vi "Acquisition Module.vi"(8 "Error In":errorcluster, 11 "Queues Cluster":T1) -> (0 "Error Out":errorcluster)   [LabVIEW 2017]
uses:
  Typedefs/Imaging Protocols enum.ctl
  User Interface/Queue/Message Queue/Typedefs/All Message Queues.ctl
  User Interface/Queue/Message Queue/Typedefs/Message Cluster.ctl
  Typedefs/Logging queue element.ctl
  Typedefs/Frame Size.ctl
  Typedefs/Acquired points count.ctl
  Video Rec Signaling/typedefs/Functions enum.ctl
  Typedefs/Read Write Enum.ctl
  Global Variables/General Globals.vi
panel:
  out "Rate":u32
  out "Acq":u32
  out "Start":u32
  out "?":errorcluster
  out "Imaging Protocol":T2=enum."Live Imaging"
  out "Acquired z-plane index":i32
  out "State":string
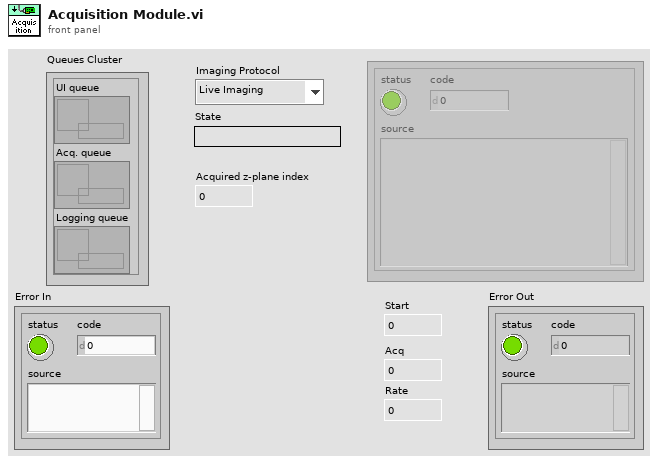
[diagram p1: front panel]
types:
  T1 = typedef "All Message Queues.ctl" = cluster{"UI queue":refnum<queue>, "Acq. queue":refnum<queue>, "Logging queue":refnum<queue>}
  T2 = typedef "Imaging Protocols enum.ctl" = enum16{"AOL Z-Stack", "Motor Z Stack", "Functional Acquisition", "Single Plane Acquisition", "Volume Acquisition", "Live Imaging", "Live Plane Imaging", "Live Volume Imaging"}
  T3 = typedef "Functions enum.ctl" = enum16{"Create", "Start", "Write", "Stop", "Clear"}
  T4 = enum8{"Enabled", "Disabled", "Disabled and Grayed Out"}
  T5 = typedef "Read Write Enum.ctl" = enum16{"Read", "Write"}
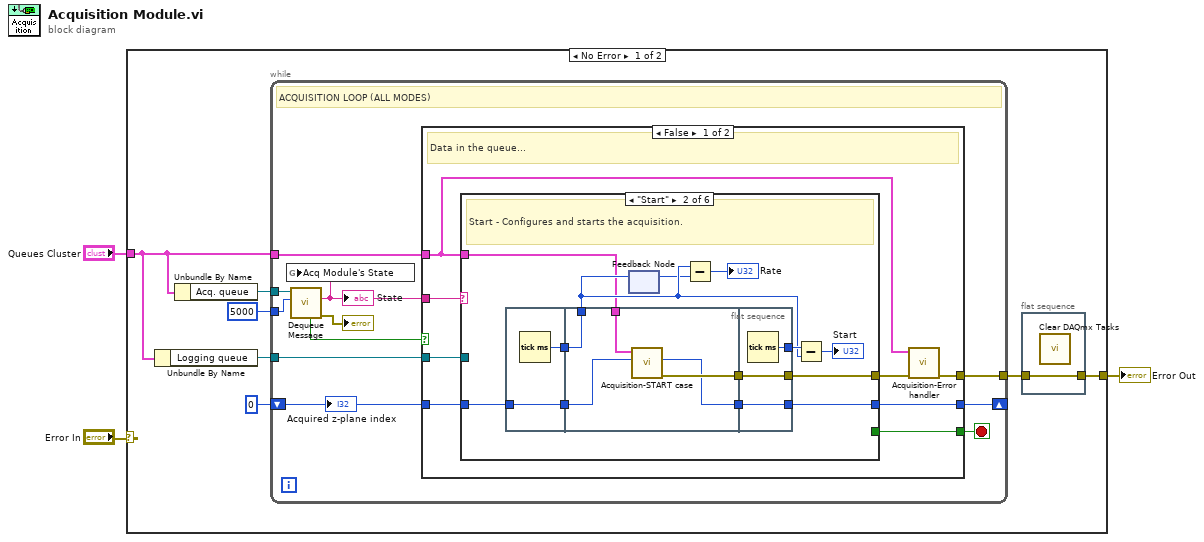
[diagram p0: block diagram]
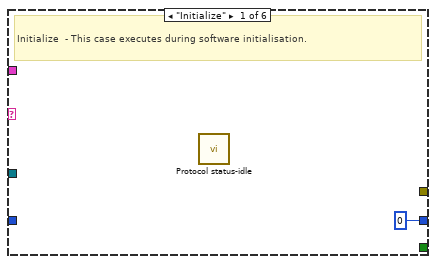
[diagram p2: hidden frame]
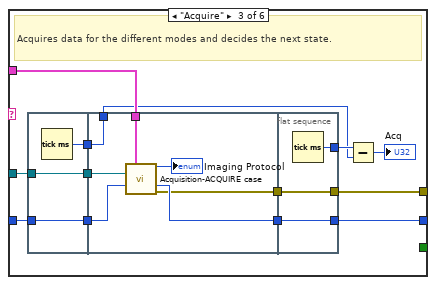
[diagram p3: hidden frame]
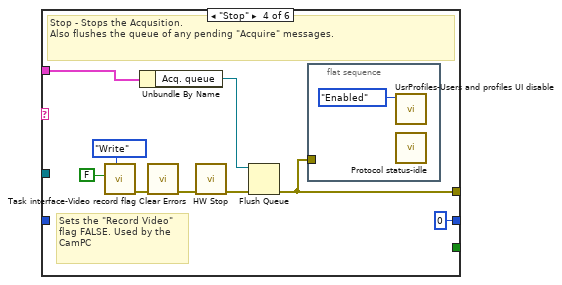
[diagram p4: hidden frame]
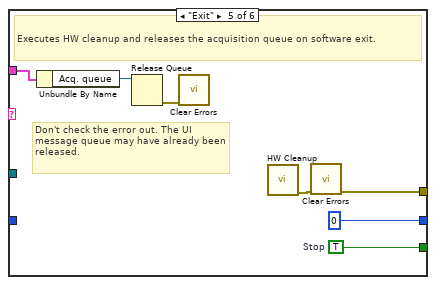
[diagram p5: hidden frame]
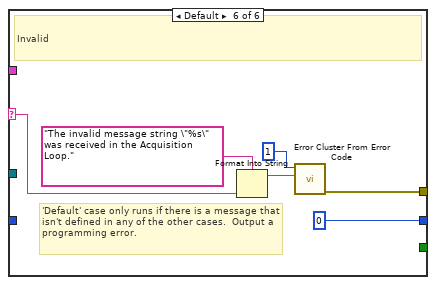
[diagram p6: hidden frame]
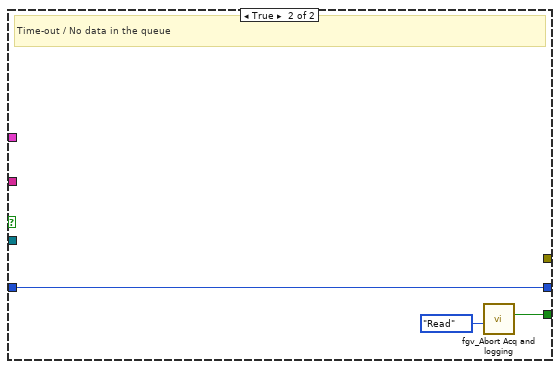
[diagram p7: hidden frame]
diagram:
  n1 = case shown="No Error" "Error In" {
    selector: "Error In" -> [_ w107]
    tunnel: "Queues Cluster" -> [w6 _]
    tunnel: [w7 w107] -> w2
    frame No Error {
      n2 = Unbundle By Name(w6) -> ("Logging queue"=w5:refnum<queue>)
      n3 = Unbundle By Name(w6) -> ("Acq. queue"=w10:refnum<queue>)
      n4 = while {
        tunnel: w10 -> [w19]
        tunnel: w5 -> [w21]
        shift-right: [w20] -> _
        shift-left: 0 -> [w18]
        tunnel: w6 -> [w17]
        tunnel: [w15] -> w8
        tunnel: 5000 ("timeout in ms (-1)") -> [w14]
        stop <- w22 stop-if-true
        # "ACQUISITION LOOP (ALL MODES)"
        n5 = call "Dequeue Message.vi"("timeout in ms (-1)"=w14, "Message Queue"=w19) -> ("Error Out"=→"?":errorcluster, "Message"=w12:string, "timed out?"=w13:bool)  [unwired: 5 in, 2 out]
        "State" <- w12
        n6 = global write "General Globals.vi" "Acq Module's State"(w12) -> ()
        n7 = case shown="False" w13 {
          tunnel: [w30 w104] -> w22
          tunnel: w21 -> [w29 _]
          tunnel: [w28 w106] -> w20
          tunnel: w18 -> [w27 w106]
          tunnel: w12 -> [w25 _]
          tunnel: w17 -> [w23 _]
          tunnel: [w24 _] -> w15
          frame False {
            # "Data in the queue..."
            n8 = case "Message Cases" shown="\"Start\"" w25 {
              selector: w25 -> [_ _ _ _ _ w99]
              tunnel: [_ w44 w64 w81 w91 w101] -> w26
              tunnel: [_ _ _ _ w97 _] -> w30
              tunnel: w29 -> [_ _ w67 _ _ _]
              tunnel: w27 -> [_ w43 w63 _ _ _]
              tunnel: [0 ("Index of next Z-plane to acquire") w42 w66 0 ("Index of next Z-plane to acquire") 0 ("Index of next Z-plane to acquire") 0 ("Index of next Z-plane to acquire")] -> w28
              tunnel: w23 -> [_ w32 w65 w82 w95 _]
              frame "Initialize" {
                # "Initialize  - This case executes during software initialisation."
                n9 = call "Protocol status-idle.vi"() -> ()  [unwired: 12 in]
              }
              frame "Start" {
                # "Start - Configures and starts the acquisition."
                n10 = flat-sequence {
                  tunnel: w43 -> [w46]
                  tunnel: [w46] -> w39
                  tunnel: [w45] -> w38
                  tunnel: w32 -> [w50]
                  tunnel: [w51] -> w41
                  tunnel: [w48] -> w40
                  tunnel: w39 -> [w49]
                  tunnel: w38 -> [w47]
                  tunnel: [w47] -> w35
                  tunnel: [w53] -> w42
                  tunnel: [w54] -> w44
                  tunnel: w41 -> [w54]
                  tunnel: w40 -> [w53]
                  tunnel: [w52] -> w37
                  frame #0 {
                    n11 = Tick Count (ms)() -> (millisecond timer value=w45:u32)
                  }
                  frame #1 {
                    n12 = call "Acquisition-START case.vi"("Acquired z-plane index"=w49, "Message Queues"=w50) -> ("error out"=w51:errorcluster, "Index of z-plane to acquire next"=w48:i32)  [unwired: 8 in]
                  }
                  frame #2 {
                    n13 = Tick Count (ms)() -> (millisecond timer value=w52:u32)
                  }
                }
                n14 = feedback-in #1(w35) -> ()
                n15 = feedback #1() -> (w34:u32)  [unwired: 1 in]
                n16 = Subtract(x=w35, y=w34) -> (x-y=→"Rate":u32)
                n17 = Subtract(x=w37, y=w35) -> (x-y=→"Start":u32)
              }
              frame "Acquire" {
                # "Acquires data for the different modes and decides the next state."
                n18 = flat-sequence {
                  tunnel: w63 -> [w69]
                  tunnel: w67 -> [w70]
                  tunnel: [w70] -> w62
                  tunnel: [w69] -> w61
                  tunnel: [w68] -> w57
                  tunnel: w65 -> [w75]
                  tunnel: w62 -> [w77]
                  tunnel: w61 -> [w73]
                  tunnel: [w76] -> w60
                  tunnel: [w74] -> w59
                  tunnel: w57 -> [w72]
                  tunnel: [w72] -> w56
                  tunnel: [w79] -> w64
                  tunnel: [w80] -> w66
                  tunnel: w60 -> [w80]
                  tunnel: w59 -> [w79]
                  tunnel: [w78] -> w58
                  frame #0 {
                    n19 = Tick Count (ms)() -> (millisecond timer value=w68:u32)
                  }
                  frame #1 {
                    n20 = call "Acquisition-ACQUIRE case.vi"("Message Queues"=w75, "Logging queue in"=w77, "Acquired z-plane index"=w73) -> ("Imaging Protocol"=→"Imaging Protocol":T2, "Index of next Z-plane to acquire"=w76:i32, "Error Out"=w74:errorcluster)  [unwired: 9 in, 1 out]
                  }
                  frame #2 {
                    n21 = Tick Count (ms)() -> (millisecond timer value=w78:u32)
                  }
                }
                n22 = Subtract(x=w58, y=w56) -> (x-y=→"Acq":u32)
              }
              frame "Stop" {
                # "Sets the \"Record Video\"\nflag FALSE. Used by the CamPC"
                # "Stop - Stops the Acqusition.\nAlso flushes the queue of any pending \"Acquire\" messages."
                n23 = call "Task interface-Video record flag.vi"("Function"=Functions_enum."Write", "DO value"=FALSE) -> ("error out"=w84:errorcluster)  [unwired: 9 in]
                n24 = Unbundle By Name(w82) -> ("Acq. queue"=w89:refnum<queue>)
                n25 = call <vilib>:"Clear Errors.vi"("error in (no error)"=w84) -> ("error out"=w86:errorcluster)  [unwired: 5 in, 1 out]
                n26 = call "HW Stop.vi"("error in (no error)"=w86) -> ("error out"=w87:errorcluster)  [unwired: 10 in]
                n27 = Flush Queue(queue=w89, error in (no error)=w87) -> (error out=w81:errorcluster)  [unwired: 2 out]
                n28 = flat-sequence {
                  tunnel: w81 -> [_]
                  frame #0 {
                    n29 = call "UsrProfiles-Users and profiles UI disable.vi"("Users & Profiles available?"=T4."Enabled") -> ()  [unwired: 10 in, 1 out]
                    n30 = call "Protocol status-idle.vi"() -> ()  [unwired: 12 in]
                  }
                }
              }
              frame "Exit" {
                w97 = TRUE  # Stop
                # "Don't check the error out. The UI message queue may have already been released."
                # "Executes HW cleanup and releases the acquisition queue on software exit."
                n31 = Unbundle By Name(w95) -> ("Acq. queue"=w96:refnum<queue>)
                n32 = Release Queue(queue=w96) -> (error out=w94:errorcluster)  [unwired: 2 in, 2 out]
                n33 = call <vilib>:"Clear Errors.vi"("error in (no error)"=w94) -> ()  [unwired: 5 in, 2 out]
                n34 = call "HW Cleanup.vi"() -> ("error out"=w92:errorcluster)  [unwired: 11 in]
                n35 = call <vilib>:"Clear Errors.vi"("error in (no error)"=w92) -> ("error out"=w91:errorcluster)  [unwired: 5 in, 1 out]
              }
              frame Default {
                # "'Default' case only runs if there is a message that isn't defined in any of the other cases.  Output a programming error."
                # "Invalid"
                n36 = Format Into String(format string="The invalid message string \"%s\" was received in the Acquisition Loop." ("Invalid Acquisition Message"), w99) -> (resulting string=w100:string)  [unwired: 2 in, 1 out]
                n37 = call <vilib>:"Error Cluster From Error Code.vi"("error message (\"\")"=w100, "error code (0)"=1) -> ("error out"=w101:errorcluster)  [unwired: 7 in]
              }
            }
            n38 = call "Acquisition-Error handler.vi"("error in (no error)"=w26, "Message Queues"=w23) -> ("error out"=w24:errorcluster)  [unwired: 9 in]
          }
          frame True {
            # "Time-out / No data in the queue"
            n39 = call "fgv_Abort Acq and logging.vi"("Function"=Read_Write_Enum."Read") -> ("Abort acquisition"=w104:bool)  [unwired: 9 in, 1 out]
          }
        }
        "Acquired z-plane index" <- w18
      }
      n40 = flat-sequence {
        tunnel: w8 -> [w11]
        tunnel: [w11] -> w7
        frame #0 {
          n41 = call "Clear DAQmx Tasks.vi"() -> ()  [unwired: 11 in, 1 out]
        }
      }
    }
    frame Error {
    }
  }
  "Error Out" <- w2
